vi "Write Roles.vi"(8 "error in (no error)":errorcluster, 10 "Roles":T1, 11 "BallPlacementAllyPlay in":refnum<class "BallPlacementAllyPlay.lvclass">) -> (0 "error out":errorcluster, 3 "BallPlacementAllyPlay out":refnum<class "BallPlacementAllyPlay.lvclass">)   [LabVIEW 2023, in "BallPlacementAllyPlay.lvclass"]
uses:
  BallPlacementAllyPlay.lvclass
  RolesBallPlacementAllyPlay.ctl
  BallPlacementEnemyRole_class/BallPlacementEnemyRole.lvclass
  BallPlacementReceiverRole_class/BallPlacementReceiverRole.lvclass
  BallPlacementPasserRole_class/BallPlacementPasserRole.lvclass
  BallPlacementAllyPlay.lvclass/BallPlacementAllyPlay.ctl
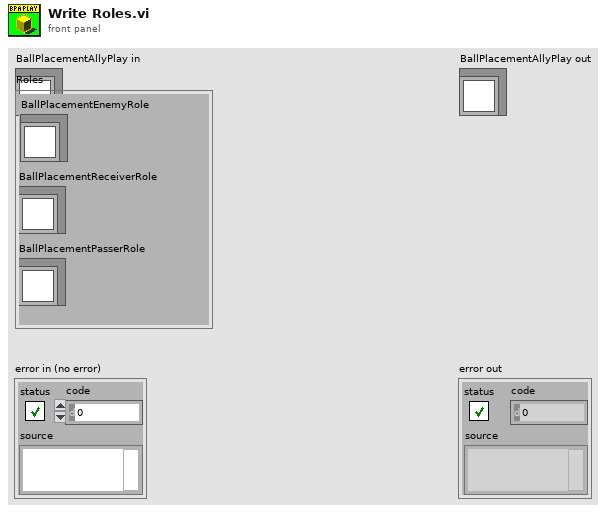
[diagram p1: front panel]
types:
  T1 = typedef "BallPlacementAllyPlay.lvclass/RolesBallPlacementAllyPlay.ctl" = cluster{"BallPlacementEnemyRole":refnum<class "BallPlacementEnemyRole.lvclass">, "BallPlacementReceiverRole":refnum<class "BallPlacementReceiverRole.lvclass">, "BallPlacementPasserRole":refnum<class "BallPlacementPasserRole.lvclass">}
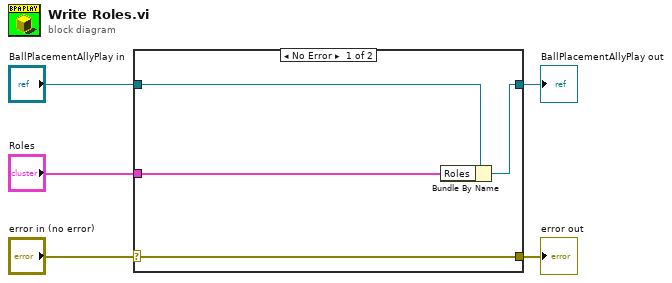
[diagram p0: block diagram]
diagram:
  n1 = case shown="No Error" "error in (no error)" {
    selector: "error in (no error)" -> [w9 w10]
    tunnel: [w9 w10] -> w4
    tunnel: [w7 w11] -> w2
    tunnel: "BallPlacementAllyPlay in" -> [w8 w11]
    tunnel: "Roles" -> [w6 _]
    frame No Error {
      n2 = Bundle By Name(cluster=w8, "Roles"=w6) -> (w7:refnum<class "BallPlacementAllyPlay.lvclass">)
    }
    frame Error {
    }
  }
  "error out" <- w4
  "BallPlacementAllyPlay out" <- w2
